vi "eps0_upd.vi"(2 "\\theta(t-1)":T1, 3 "error in (no error)":errorcluster, 4 "y(t)":dbl, 5 "\\phi(t)":T1) -> (0 "error out":errorcluster, 1 "\\eps_o(t)":dbl)   [LabVIEW 2021]
uses:
  <vilib>/Analysis/Matrix/Datatypes/RealMatrix.ctl
  <vilib>/Analysis/Matrix/Numeric/Multiply/Multiply - RM,RM.vi
  <vilib>/Analysis/Matrix/NI_Matrix.lvlib
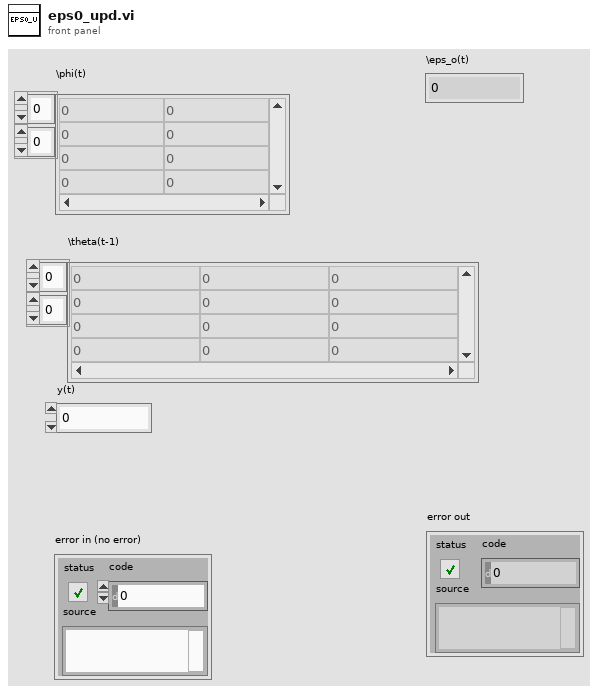
[diagram p1: front panel]
types:
  T1 = typedef "NI_Matrix.lvlib/RealMatrix.ctl" = dbl[][]
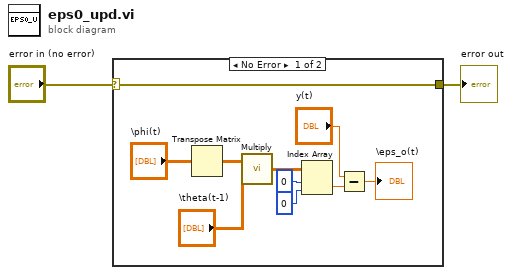
[diagram p0: block diagram]
diagram:
  n1 = case shown="No Error" "error in (no error)" {
    selector: "error in (no error)" -> [w9 w13]
    tunnel: [w9 w13] -> w1
    frame No Error {
      n2 = Transpose Matrix(1:"\\phi(t)") -> (0:w10:T1)
      n3 = call-poly <vilib>:"Multiply.vi"("Real Matrix B"="\\theta(t-1)", "Real Matrix A"=w10) -> ("A * B"=w5:T1)
      n4 = Index Array(array=w5, index (row)=0, index (col)=0) -> (element=w4:dbl)
      n5 = Subtract ("Subtract.vi")(x="y(t)", y=w4) -> (x-y=→"\\eps_o(t)":dbl)
    }
    frame Error {
    }
  }
  "error out" <- w1
